vi "Common PS UINT8 to Boolean.vi"(8 "error in (no error)":errorcluster, 10 "PS Matrix Mapping":cluster{u32[]}[](array[cluster]), 11 "PS Status (per PS Rack)":u8[](array[numeric])) -> (0 "error out":errorcluster, 3 "PS Status":bool[](array[boolean]))   [LabVIEW 2011, in "Common VIs.lvlib"]
doc: "Decode the digital I/O of all Actuation Chassis from byte representation to a vector of boolean values ordered with the same indexes as the Response Matrix columns."
uses:
  Common VIs.lvlib
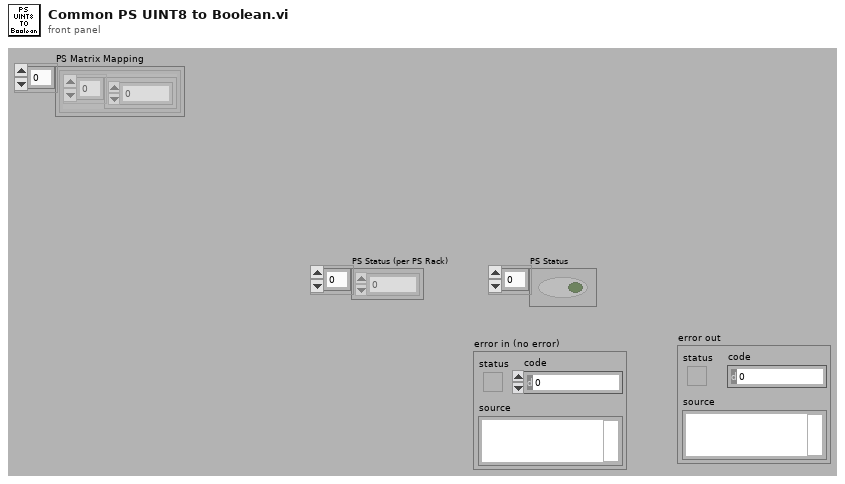
[diagram p1: front panel]
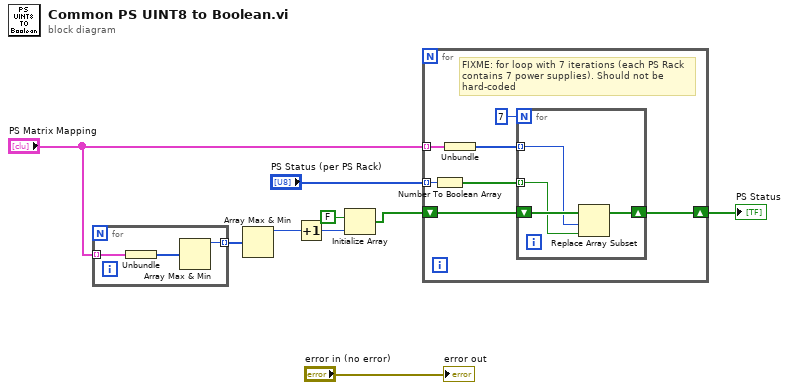
[diagram p0: block diagram]
diagram:
  n1 = for {
    tunnel: "PS Matrix Mapping" -> [w12] mode=indexing
    tunnel: [w10] -> w2 mode=indexing
    n2 = Unbundle(w12) -> (w11:u32[])
    n3 = Array Max & Min(array=w11) -> (max value=w10:u32)  [unwired: 3 out]
  }
  n4 = Array Max & Min(array=w2) -> (max value=w1:u32)  [unwired: 3 out]
  n5 = Increment(x=w1) -> (x+1=w4:u32)
  n6 = Initialize Array(FALSE, w4) -> (w6:bool[])
  n7 = for {
    tunnel: "PS Status (per PS Rack)" -> [w19] mode=indexing
    tunnel: "PS Matrix Mapping" -> [w14] mode=indexing
    shift-right: [w16] -> w9
    shift-left: w6 -> [w17]
    # "FIXME: for loop with 7 iterations (each PS Rack contains 7 power supplies). Should not be hard-coded"
    n8 = Number To Boolean Array(number=w19) -> (Boolean array=w18:bool[])
    n9 = Unbundle(w14) -> (w13:u32[])
    n10 = for {
      N: 7 -> [_]
      tunnel: w13 -> [w22] mode=indexing
      tunnel: w18 -> [w21] mode=indexing
      shift-right: [w20] -> w16
      shift-left: w17 -> [w23]
      n11 = Replace Array Subset(array=w23, new element=w21, index=w22) -> (w20:bool[])
    }
  }
  "PS Status" <- w9
  "error out" <- "error in (no error)"
